vi "trivial_req.vi"() -> ()   [LabVIEW 2014]
uses:
  lvnanomsg/nanomsg_context.lvclass
  lvnanomsg/nanomsg_socket.lvclass
panel:
  out "reply":string
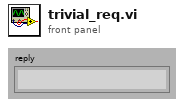
[diagram p1: front panel]
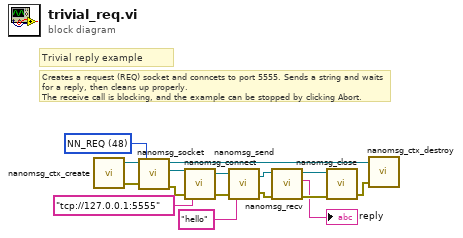
[diagram p0: block diagram]
diagram:
  w3 = 48 items=["NN_WS"=-4, "NN_TCP"=-3, "NN_IPC"=-2, "NN_INPROC"=-1, "NN_SOL_SOCKET"=0, "NN_PAIR"=16, "NN_PUB"=32, "NN_SUB"=33, "NN_REQ"=48, "NN_REP"=49, "NN_PUSH"=80, "NN_PULL"=81, "NN_SURVEYOR"=98, "NN_RESPONDENT"=99, "NN_BUS"=112] ("socket type")
  # "Creates a request (REQ) socket and conncets to port 5555. Sends a string and waits for a reply, then cleans up properly.\nThe receive call is blocking, and the example can be stopped by clicking Abort."
  # "Trivial reply example"
  n1 = call "nanomsg_ctx_create.vi"() -> ("error out"=w6:errorcluster, "context out"=w16:refnum<class "nanomsg_context.lvclass">)  [unwired: 4 in]
  n2 = call "nanomsg_socket.vi"("error in"=w6, "socket type"=w3, "context in"=w16) -> ("error out"=w15:errorcluster, "socket out"=w14:refnum<class "nanomsg_socket.lvclass">, "context out"=w7:refnum<class "nanomsg_context.lvclass">)  [unwired: 2 in]
  n3 = call "nanomsg_connect.vi"("error in"=w15, "endpoint"="tcp://127.0.0.1:5555", "socket in"=w14) -> ("error out"=w13:errorcluster, "socket out"=w12:refnum<class "nanomsg_socket.lvclass">)  [unwired: 1 in]
  n4 = call "nanomsg_send.vi"("error in"=w13, "data"="hello", "socket in"=w12) -> ("error out"=w5:errorcluster, "socket out"=w11:refnum<class "nanomsg_socket.lvclass">)  [unwired: 1 in]
  n5 = call "nanomsg_recv.vi"("error in"=w5, "socket in"=w11) -> ("error out"=w10:errorcluster, "data"=→"reply":string, "socket out"=w9:refnum<class "nanomsg_socket.lvclass">)  [unwired: 3 in, 2 out]
  n6 = call "nanomsg_close.vi"("error in"=w10, "socket"=w9) -> ("error out"=w8:errorcluster)  [unwired: 3 in]
  n7 = call "nanomsg_ctx_destroy.vi"("error in"=w8, "context in"=w7) -> ()  [unwired: 3 in, 1 out]
